vi "Read navX Registry Cache.vi"(8 "error in (no error)":errorcluster, 11 "navX - Base in":refnum<class "navX - Base.lvclass">) -> (0 "error out":errorcluster, 2 "navX Library v3.lvlib:navX Registry Cache.lvclass":refnum<class "navX Registry Cache.lvclass">, 3 "navX - Base out":refnum<class "navX - Base.lvclass">)   [LabVIEW 2015, in "navX Library v3.lvlib" / "navX - Base.lvclass"]
uses:
  navX - Base.lvclass
  navX Registry Cache/navX Registry Cache.lvclass
  navX - Base.lvclass/navX - Base.ctl
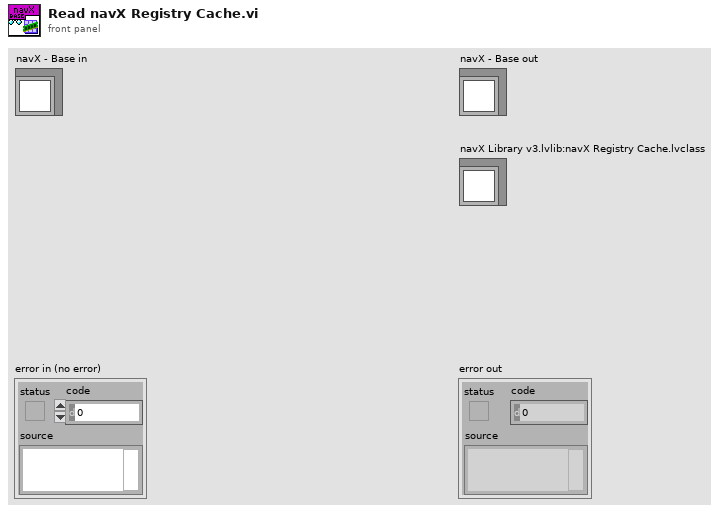
[diagram p1: front panel]
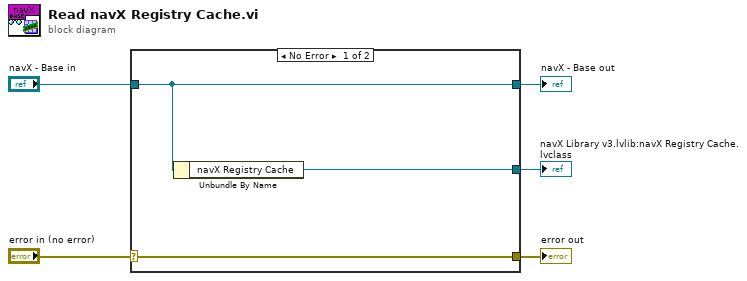
[diagram p0: block diagram]
diagram:
  n1 = case shown="No Error" "error in (no error)" {
    selector: "error in (no error)" -> [w8 w9]
    tunnel: [w8 w9] -> w4
    tunnel: [w7 w10] -> w2
    tunnel: "navX - Base in" -> [w7 w10]
    tunnel: [w6 _] -> w1
    frame No Error {
      n2 = Unbundle By Name(w7) -> ("navX Registry Cache"=w6:refnum<class "navX Registry Cache.lvclass">)
    }
    frame Error {
    }
  }
  "error out" <- w4
  "navX - Base out" <- w2
  "navX Library v3.lvlib:navX Registry Cache.lvclass" <- w1
